vi "GenerateDiverageGrid.vi"(2 "俯仰CCD0":dbl, 3 "TargetTheta":dbl, 4 "旋转CCD0":dbl, 5 "L":dbl) -> (0 "PitchGrid":dbl[](array[numeric]), 1 "RollGrid":dbl[](array[numeric]))   [LabVIEW 2018]
panel:
  # "计算当前位置发散角点阵\n输入当前位置L和计算位置TargetTheta\n还需要加入ccd0位置时的角度"
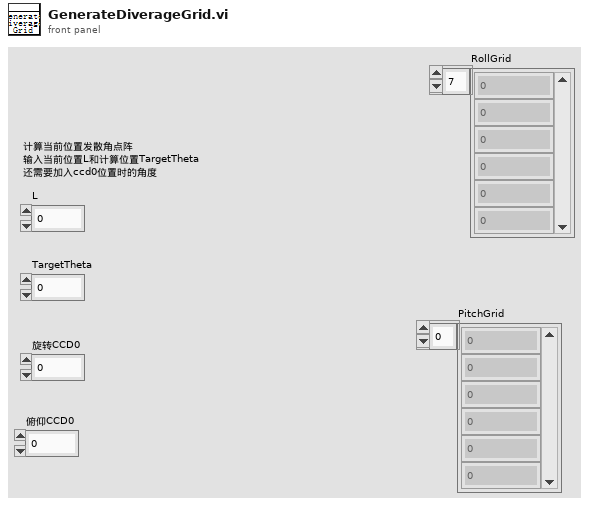
[diagram p1: front panel]
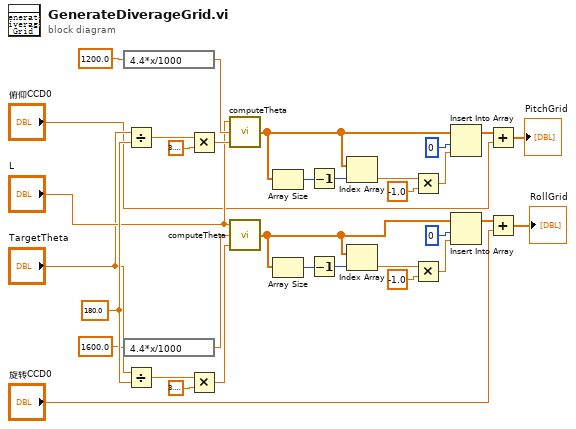
[diagram p0: block diagram]
diagram:
  w30 = 180.0 ("y")
  n1 = expression code="4.4*x/1000"(1200.0) -> (w23:dbl)
  n2 = expression code="4.4*x/1000"(1600.0) -> (w24:dbl)
  n3 = Divide(x="TargetTheta", y=w30) -> (x/y=w29:dbl)
  n4 = Divide(x="TargetTheta", y=w30) -> (x/y=w33:dbl)
  n5 = Multiply(x=w29, y=3.141592653589793) -> (x*y=w27:dbl)
  n6 = Multiply(x=w33, y=3.141592653589793) -> (x*y=w31:dbl)
  n7 = call "computeTheta.vi"("thetaT"=w27, "M"=w23, "L"="L") -> ("ThetaOut"=w8:dbl[])  [unwired: 2 in]
  n8 = call "computeTheta.vi"("thetaT"=w31, "M"=w24, "L"="L") -> ("ThetaOut"=w20:dbl[])  [unwired: 2 in]
  n9 = Array Size(array=w8) -> (size(s)=w13:i32)
  n10 = Array Size(array=w20) -> (size(s)=w19:i32)
  n11 = Decrement(x=w13) -> (x-1=w12:i32)
  n12 = Decrement(x=w19) -> (x-1=w18:i32)
  n13 = Index Array(array=w8, index=w12) -> (element=w11:dbl)
  n14 = Index Array(array=w20, index=w18) -> (element=w17:dbl)
  n15 = Multiply(x=w11, y=-1.0) -> (x*y=w9:dbl)
  n16 = Multiply(x=w17, y=-1.0) -> (x*y=w15:dbl)
  n17 = Insert Into Array(array=w8, index=0, new element=w9) -> (w3:dbl[])
  n18 = Insert Into Array(array=w20, index=0, new element=w15) -> (w6:dbl[])
  n19 = Add(x=w3, y="俯仰CCD0") -> (x+y=→"PitchGrid":dbl[])
  n20 = Add(x=w6, y="旋转CCD0") -> (x+y=→"RollGrid":dbl[])
